vi "Test Main.vi"() -> ()   [LabVIEW 2017]
uses:
  Implementation/Git Implementation.lvclass
  Implementation/Reset Mode.ctl
  Implementation/Add Options.ctl
panel:
  out "Status Messages":string[](array[string])
  out "error out":errorcluster
  in  "Remote URL":string="git@github.com:oist/Chakraborty_FanucNSProxy"
  in  "Target Directory":path=path "C:/Users/Christian/Desktop/junk-test-git-dir"
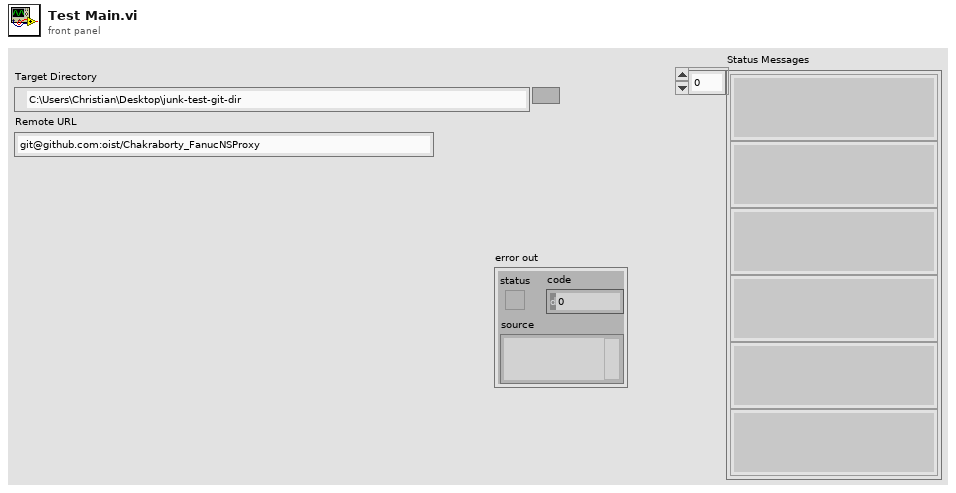
[diagram p1: front panel]
types:
  T1 = typedef "Git Implementation.lvclass/Add Options.ctl" = cluster{"All":bool, "Force":bool, "Continue on Error":bool, "Intent Only":bool}
  T2 = typedef "Git Implementation.lvclass/Reset Mode.ctl" = enum16{"mixed", "soft", "hard", "merge", "keep"}
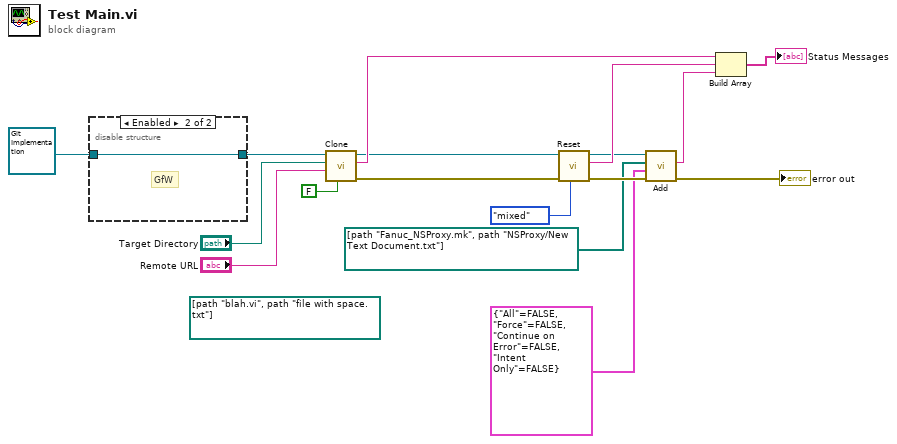
[diagram p0: block diagram]
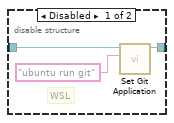
[diagram p2: hidden frame]
diagram:
  (unwired) path[] [path "blah.vi", path "file with space.txt"] ("Files to Reset")
  n1 = disable-structure shown="Enabled" {
    disable-tunnel: refnum<class "Git Implementation.lvclass"> refnum ("Git Implementation.lvclass") -> [w20 w21]
    disable-tunnel: [w19 w21] -> w15
    frame Disabled {
      # "WSL"
      n2 = call "Set Git Application.vi"("Git Application"="ubuntu run git", "Git Implementation in"=w20) -> ("Git Implementation out"=w19:refnum<class "Git Implementation.lvclass">)  [unwired: 9 in]
    }
    frame Enabled {
      # "GfW"
    }
  }
  n3 = call "Clone.vi"("Error on existing directory"=FALSE, "Remote URL"="Remote URL", "Target Directory"="Target Directory", "Git Implementation in"=w15) -> ("error out"=w12:errorcluster, "Status Message"=w17:string, "Git Implementation out"=w9:refnum<class "Git Implementation.lvclass">)  [unwired: 5 in]
  n4 = call "Reset.vi"("Reset Mode"=Reset_Mode."mixed", "error in (no error)"=w12, "Git Implementation in"=w9) -> ("error out"=w6:errorcluster, "Status Message"=w7:string, "Git Implementation out"=w4:refnum<class "Git Implementation.lvclass">)  [unwired: 6 in]
  n5 = call "Add.vi"("error in (no error)"=w6, "Add Options"=T1 {"All"=FALSE, "Force"=FALSE, "Continue on Error"=FALSE, "Intent Only"=FALSE}, "Files to Add"=path[] [path "Fanuc_NSProxy.mk", path "NSProxy/New Text Document.txt"], "Git Implementation in"=w4) -> ("error out"=→"error out":errorcluster, "Status Message"=w3:string)  [unwired: 5 in, 1 out]
  n6 = Build Array(w17, w7, w3) -> (→"Status Messages":string[])
